vi "Fpga-2-U64-to-U8-Array.vi"(10 "Numeric":u64, 11 "Numeric 2":u64) -> (3 "Array":u8[](array[numeric]))   [LabVIEW 2017]
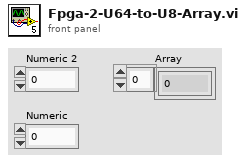
[diagram p1: front panel]
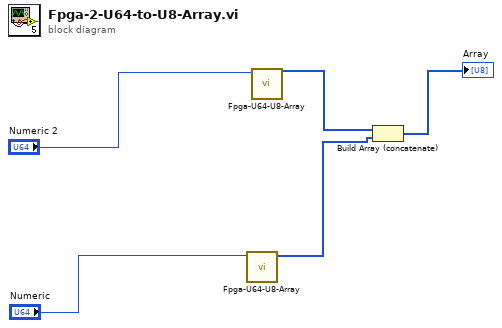
[diagram p0: block diagram]
diagram:
  n1 = call "Fpga-U64-U8-Array.vi"("Numeric"="Numeric") -> ("Array"=w4:u8[])  [unwired: 10 in]
  n2 = call "Fpga-U64-U8-Array.vi"("Numeric"="Numeric 2") -> ("Array"=w3:u8[])  [unwired: 10 in]
  n3 = Build Array (concatenate)(w3, w4) -> (→"Array":u8[])
